vi "LV SciSDK OSCILLOSCOPE DUAL GET STATUS.vi"(7 "Oscilloscope Handle In":T3, 9 "Board Handle In":T1, 11 "error in (no error)":errorcluster) -> (4 "NI Error Code":i32, 6 "Oscilloscope Status Out":T2, 8 "Oscilloscope Handle Out":T3, 10 "Board Handle Out":T1, 15 "error out":errorcluster)   [LabVIEW 2021, in "SciSDK_Labview.lvlib"]
uses:
  SciSDK_Labview.lvlib
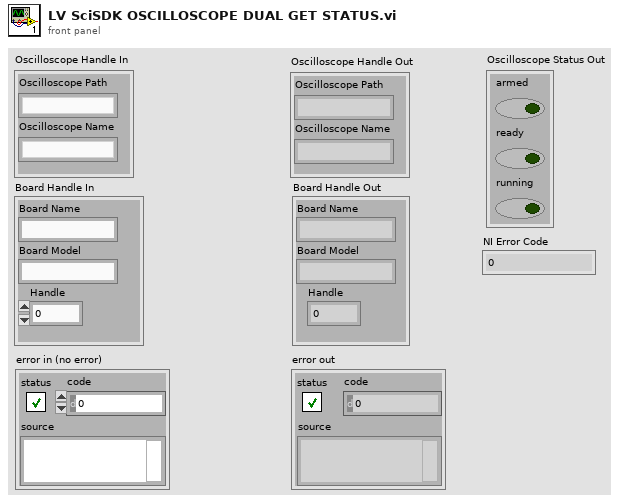
[diagram p1: front panel]
types:
  T1 = cluster{"Board Name":string, "Board Model":string, "Handle":u64}
  T2 = cluster{"armed":bool, "ready":bool, "running":bool}
  T3 = cluster{"Oscilloscope Path":string, "Oscilloscope Name":string}
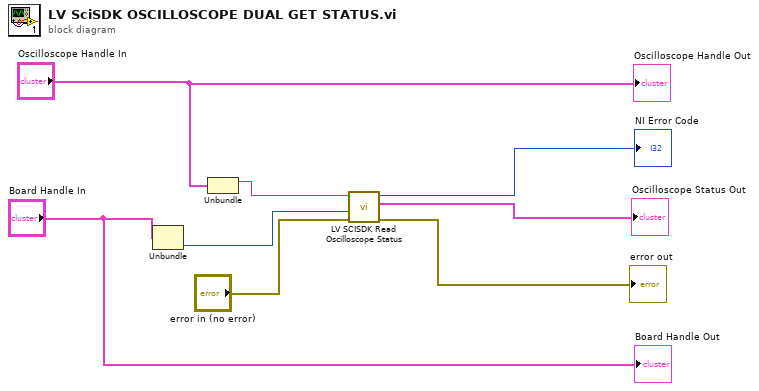
[diagram p0: block diagram]
diagram:
  n1 = Unbundle("Board Handle In") -> ("Handle"=w1:u64)  [unwired: 2 out]
  n2 = Unbundle("Oscilloscope Handle In") -> ("Oscilloscope Path"=w3:string)  [unwired: 1 out]
  n3 = call "LV SCISDK Read Oscilloscope Status.vi"("Path"=w3, "handle"=w1, "error in (no error)"="error in (no error)") -> ("function return"=→"NI Error Code":i32, "buffer out"=→"Oscilloscope Status Out":T2, "error out"=→"error out":errorcluster)  [unwired: 4 in, 1 out]
  "Oscilloscope Handle Out" <- "Oscilloscope Handle In"
  "Board Handle Out" <- "Board Handle In"
